vi "WinConditionsNumeric.vi"(11 "NumericGameboard":i8[](array[numeric])) -> (2 "LineIndices":i8[](array[numeric]), 3 "End?":bool)   [LabVIEW 2020]
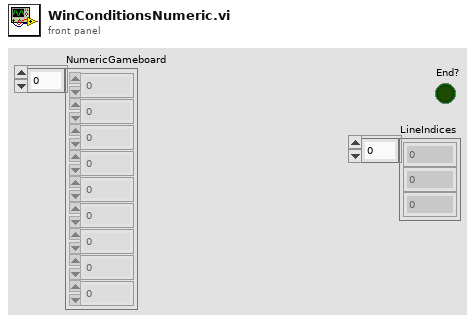
[diagram p1: front panel]
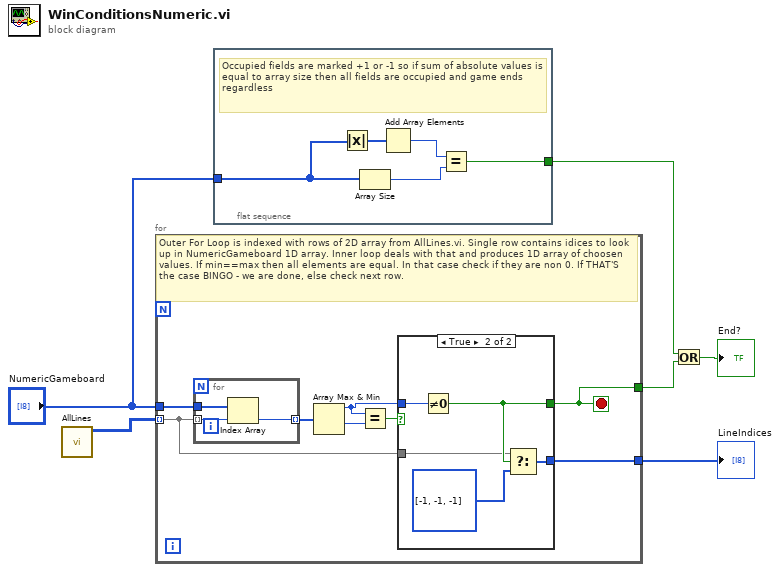
[diagram p0: block diagram]
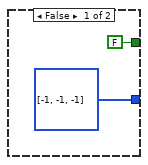
[diagram p2: hidden frame]
diagram:
  n1 = call "AllLines.vi"() -> ("Lines"=w6:i8[][])  [unwired: 11 in]
  n2 = for {
    tunnel: w6 -> [w9] mode=indexing
    tunnel: "NumericGameboard" -> [w14]
    tunnel: [w8] -> w3
    tunnel: [w7] -> w5
    stop <- w8 stop-if-true
    # "Outer For Loop is indexed with rows of 2D array from AllLines.vi. Single row contains idices to look up in NumericGameboard 1D array. Inner loop deals with that and produces 1D array of choosen values. If min==max then all elements are equal. In that case check if they are non 0. If THAT'S the case BINGO - we are done, else check next row."
    n3 = for {
      tunnel: w14 -> [w24]
      tunnel: w9 -> [w23] mode=indexing
      tunnel: [w22] -> w13 mode=indexing
      n4 = Index Array(array=w24, index=w23) -> (element=w22:i8)
    }
    n5 = Array Max & Min(array=w13) -> (max value=w10:i8, min value=w12:i8)  [unwired: 2 out]
    n6 = Equal?(x=w10, y=w12) -> (x = y?=w11:bool)
    n7 = case shown="True" w11 {
      tunnel: w10 -> [_ w21]
      tunnel: w9 -> [_ w18]
      tunnel: [FALSE w19] -> w8
      tunnel: [i8[] [-1, -1, -1] ("Lines") w20] -> w7
      frame False {
      }
      frame True {
        n8 = Not Equal To 0?(x=w21) -> (x != 0?=w19:bool)
        n9 = Select(t=w18, s=w19, f=i8[] [-1, -1, -1] ("Lines")) -> (s? t:f=w20:i8[])
      }
    }
  }
  "LineIndices" <- w5
  n10 = flat-sequence {
    tunnel: "NumericGameboard" -> [w26]
    tunnel: [w25] -> w2
    frame #0 {
      # "Occupied fields are marked +1 or -1 so if sum of absolute values is equal to array size then all fields are occupied and game ends regardless"
      n11 = Absolute Value(x=w26) -> (abs(x)=w28:i8[])
      n12 = Array Size(array=w26) -> (size(s)=w29:i32)
      n13 = Add Array Elements(numeric array=w28) -> (sum=w27:i8)
      n14 = Equal?(x=w27, y=w29) -> (x = y?=w25:bool)
    }
  }
  n15 = Or(x=w2, y=w3) -> (x .or. y?=→"End?":bool)
